vi "zad1.vi"() -> ()   [LabVIEW 2017]
uses:
  <vilib>/sound2/lvsound2.llb/Sound Input Read (DBL).vi
  <vilib>/sound2/lvsound2.llb/Sound Data Format.ctl
  <vilib>/sound2/lvsound2.llb/Sampling Mode.ctl
panel:
  out "Power Spectrum":cluster{"f0":dbl, "df":dbl, "magnitude":dbl[]}[](graph)
  out "Waveform Graph":waveform(dbl)[](graph)
  in  "stop":bool
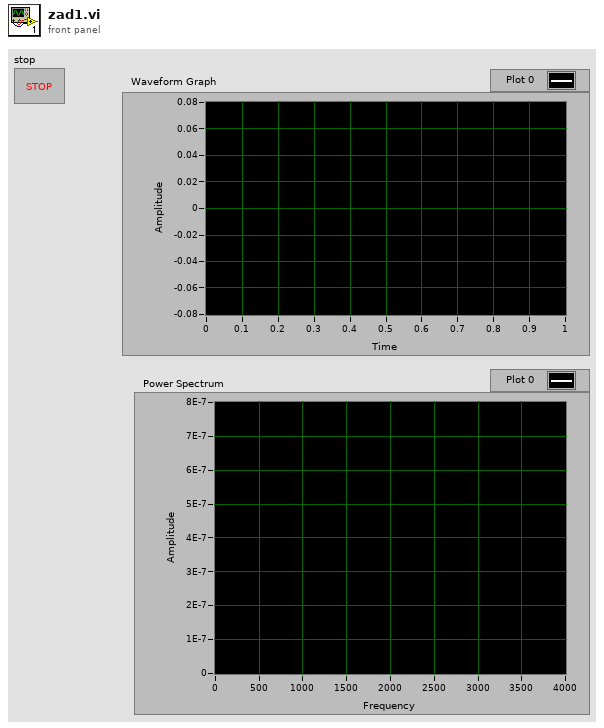
[diagram p1: front panel]
types:
  T1 = typedef "Sampling Mode.ctl" = i32
  T2 = typedef "Sound Data Format.ctl" = cluster{"sample rate (S/s)":dbl, "number of channels":i32, "bits per sample":i32}
  T3 = typedef "Sound Input Task ID.ctl" = u32
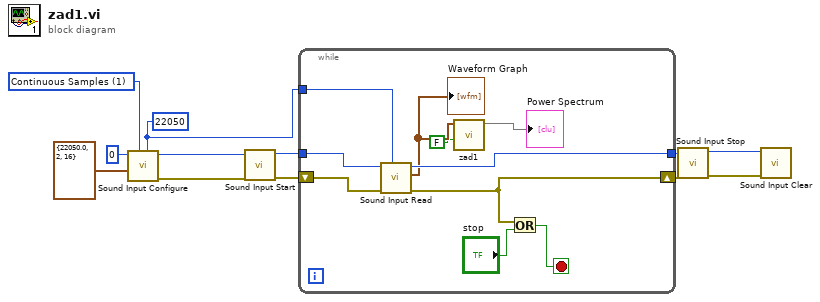
[diagram p0: block diagram]
diagram:
  w4 = T1 1 items=["Finite Samples", "Continuous Samples"] ("sample mode")
  w1 = 22050 ("number of samples/ch")
  n1 = call <vilib>:"Sound Input Configure.vi"("number of samples/ch"=w1, "sample mode"=w4, "sound format"=T2 {"sample rate (S/s)"=22050.0, "number of channels"=2, "bits per sample"=16}, "device ID"=u32 0) -> ("error out"=w11:errorcluster, "task ID"=w6:T3)  [unwired: 6 in]
  n2 = call <vilib>:"Sound Input Start.vi"("error in (no error)"=w11, "task ID"=w6) -> ("error out"=w10:errorcluster, "task ID out"=w5:T3)  [unwired: 8 in]
  n3 = while {
    tunnel: w5 -> [w21]
    tunnel: w1 -> [w20]
    shift-right: [w18] -> w9
    shift-left: w10 -> [w22]
    tunnel: [w16] -> w3
    stop <- w17 stop-if-true
    n4 = call-poly <vilib>:"Sound Input Read.vi"("number of samples/ch"=w20, "error in (no error)"=w22, "task ID"=w21) -> ("error out"=w18:errorcluster, "data"=w15:waveform(dbl)[], "task ID out"=w16:T3)  [unwired: 6 in]
    "Waveform Graph" <- w15
    n5 = call "zad1.vi"(9:FALSE ("dB On (T)"), 11:w15) -> (3:→"Power Spectrum")  [unwired: 9 in]
    n6 = Or(x=w18, y="stop") -> (x .or. y?=w17:bool)
  }
  n7 = call <vilib>:"Sound Input Stop.vi"("error in (no error)"=w9, "task ID"=w3) -> ("error out"=w8:errorcluster, "task ID out"=w2:T3)  [unwired: 8 in]
  n8 = call <vilib>:"Sound Input Clear.vi"("error in (no error)"=w8, "task ID"=w2) -> ()  [unwired: 9 in, 1 out]
